vi "Create.vi"(6 "Labels":map{string, string}(c390), 7 "Registry Name":string="_default_registry", 8 "error in (no error)":errorcluster, 9 "Auto-register?":bool=TRUE, 10 "Description":string, 11 "Metric Name":string) -> (0 "error out":errorcluster, 3 "Gauge Ref":refnum<data-value>)   [LabVIEW 2020, in "Metrics.lvlib" / "Gauge.lvclass"]
uses:
  Gauge.lvclass
  C:/Github-locals/PromVIEW/src/metrics/metric/Metric.lvclass
  metric/Metric.lvclass/Metric.ctl
  metric/Write Name.vi
  metric/Write Description.vi
  metric/Validate Name.vi
  registry/session/Registry Session.lvclass
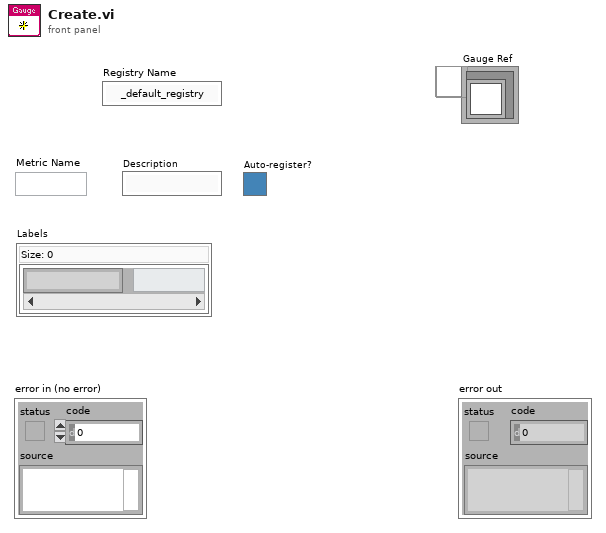
[diagram p1: front panel]
types:
  T1 = typedef "Registry.lvlib/Registry Session.lvclass/Session Handle.ctl" = refnum<data-value>
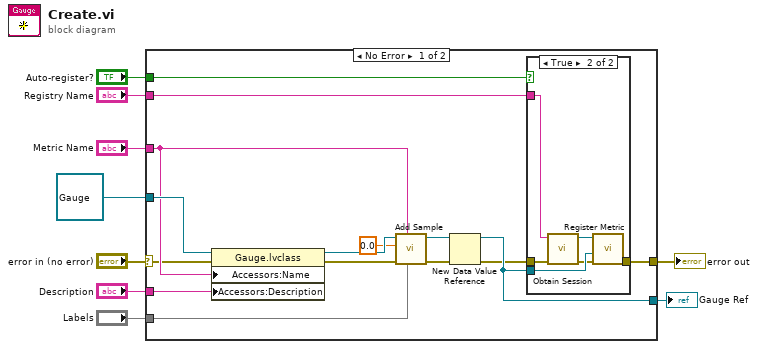
[diagram p0: block diagram]
diagram:
  n1 = case shown="No Error" "error in (no error)" {
    selector: "error in (no error)" -> [w10 w32]
    tunnel: [w16 w32] -> w8
    tunnel: "Metric Name" -> [w15 _]
    tunnel: "Labels" -> [w18 _]
    tunnel: "Description" -> [w23 _]
    tunnel: refnum<class "Gauge.lvclass"> refnum ("Metrics.lvlib:Gauge.lvclass") -> [w24 _]
    tunnel: [w14 _] -> w1
    tunnel: "Registry Name" -> [w17 _]
    tunnel: "Auto-register?" -> [w12 _]
    frame No Error {
      n2 = property class="Gauge.lvclass"(reference=w24, error in=w10, "Accessors:Name"=w15, "Accessors:Description"=w23) -> (reference out=w22:refnum<class "Gauge.lvclass">, error out=w11:errorcluster)
      n3 = call-dynamic "Add Sample.vi"("Labels"=w18, "Sample Name"=w15, "error in (no error)"=w11, "Value"=0.0, "Metric in"=w22) -> ("error out"=w19:errorcluster, "Metric out"=w20:refnum<class "Gauge.lvclass">)  [unwired: 5 in]
      n4 = New Data Value Reference(data value=w20, error in=w19) -> (data value reference=w14:refnum<data-value>, error out=w13:errorcluster)
      n5 = case shown="True" w12 {
        tunnel: w17 -> [_ w31]
        tunnel: [w25 w30] -> w16
        tunnel: w14 -> [_ w29]
        tunnel: w13 -> [w25 w27]
        frame False {
        }
        frame True {
          n6 = call "Obtain Session.vi"("error in (no error)"=w27, "Session  Name ()"=w31) -> ("error out"=w26:errorcluster, "Session Handle"=w28:T1)  [unwired: 8 in]
          n7 = call "Register Metric.vi"("error in (no error)"=w26, "New Metric"=w29, "Session Handle in"=w28) -> ("error out"=w30:errorcluster)  [unwired: 7 in, 1 out]
        }
      }
    }
    frame Error {
    }
  }
  "error out" <- w8
  "Gauge Ref" <- w1
